vi "ARCH_AUDIT_EDITOR_prepare_SELECT_statement.vi"(7 "nmb_of_top_rows (all)":i32, 8 "error_in":errorcluster) -> (0 "error_out":errorcluster, 3 "SELECT_statement":string)   [LabVIEW 2020]
uses:
  FGV/ARCH_AUDIT_EDITOR_records_display/FGV_ARCH_AUDIT_EDITOR_records_display.ctl
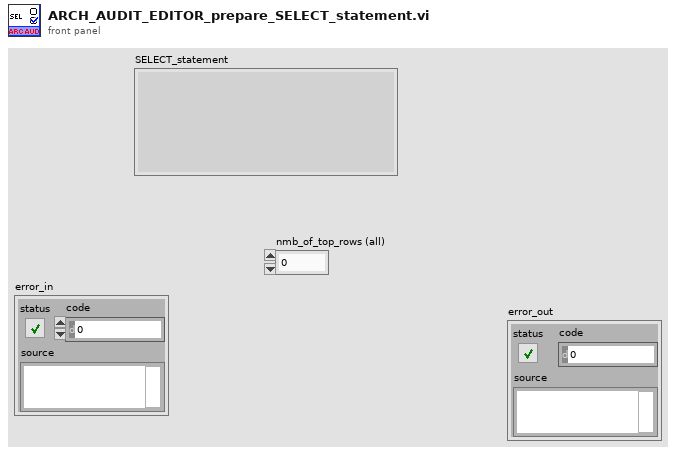
[diagram p1: front panel]
types:
  T1 = typedef "FGV_ARCH_AUDIT_EDITOR_records_display.ctl" = enum16{"initialize", "set_arch_cfg_tables_names", "set_station_number", "set_type_filter", "set_headers", "set_records", "get_arch_cfg_table_name", "get_arch_cfg_hist_table_name", "get_station_number", "get_type_filter", "get_headers", "get_uneditable_columns", "get_all_info", "record_added?", "record_inserted?", "record_edited?", "record_updated?", "record_deleted?", "discard_changes"}
  T2 = typedef "ARCH_AUDIT_EDITOR_all_info.ctl" = cluster{"station_number":string, "type_filter":string, "archivisation_audit_cfg_table":string, "archivisation_audit_cfg_history":string, "column_names":string[], "uneditable_columns":string[], "uneditable_columns":i32[], "editable_columns":i32[], "values_in_database":string[][], "size":cluster{"columns":i32, "SQL_rows":i32, "disp_rows":i32}, "ARCH_AUDIT_record_states":T3[]}
  T3 = typedef "SQL_record_states.ctl" = enum16{"Equal", "Added", "Edited", "Deleted"}
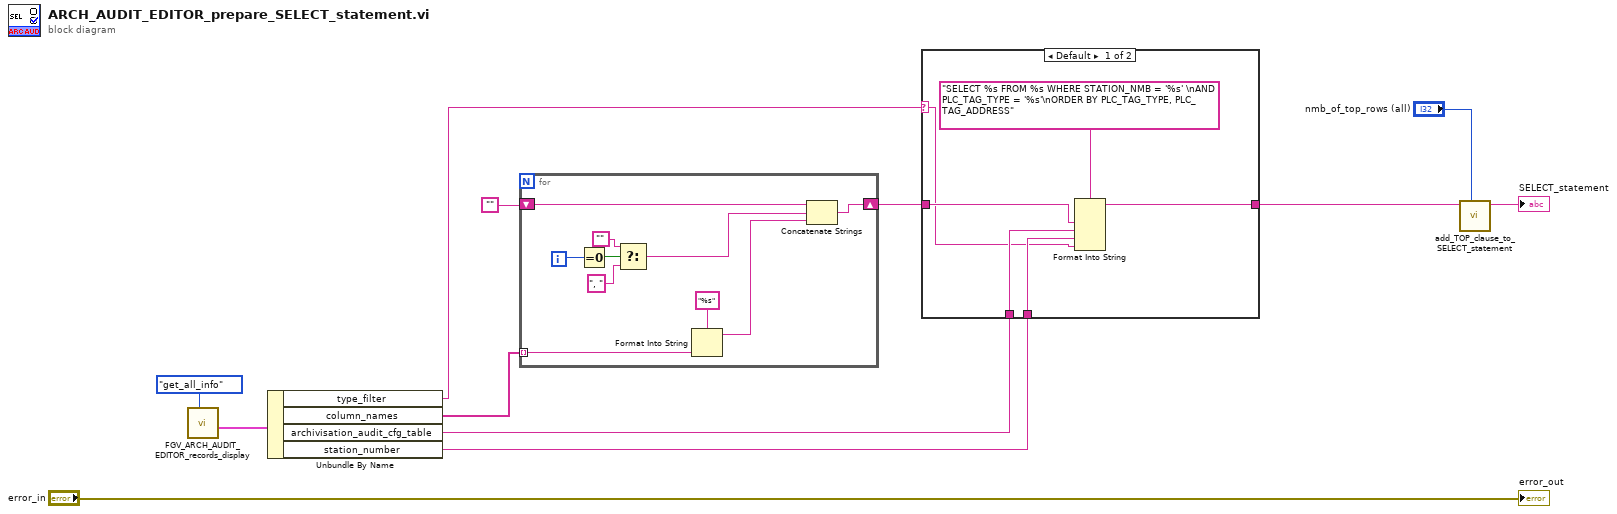
[diagram p0: block diagram]
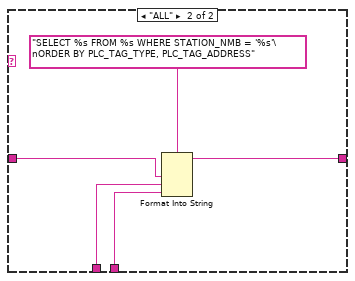
[diagram p2: hidden frame]
diagram:
  n1 = call "FGV_ARCH_AUDIT_EDITOR_records_display.vi"("options"=FGV_ARCH_AUDIT_EDITOR_records_display."get_all_info") -> ("all_info"=w5:T2)  [unwired: 7 in, 3 out]
  n2 = Unbundle By Name(w5) -> ("type_filter"=w7:string, "column_names"=w12:string[], "archivisation_audit_cfg_table"=w9:string, "station_number"=w8:string)
  n3 = for {
    tunnel: w12 -> [w15] mode=indexing
    shift-right: [w17] -> w10
    shift-left: "" -> [w18]
    i -> [w22]
    n4 = Equal To 0?(x=w22) -> (x = 0?=w21:bool)
    n5 = Select(t="", s=w21, f=", ") -> (s? t:f=w16:string)
    n6 = Format Into String(format string="%s", w15) -> (resulting string=w14:string)  [unwired: 2 in, 1 out]
    n7 = Concatenate Strings(w18, w16, w14) -> (w17:string)
  }
  n8 = case shown="Default" w7 {
    selector: w7 -> [w23 _]
    tunnel: w10 -> [w27 w32]
    tunnel: w9 -> [w25 w31]
    tunnel: w8 -> [w24 w30]
    tunnel: [w26 w29] -> w3
    frame Default {
      n9 = Format Into String(format string="SELECT %s FROM %s WHERE STATION_NMB = '%s' \nAND PLC_TAG_TYPE = '%s'\nORDER BY PLC_TAG_TYPE, PLC_TAG_ADDRESS", w27, w25, w24, w23) -> (resulting string=w26:string)  [unwired: 2 in, 1 out]
    }
    frame "ALL" {
      n10 = Format Into String(format string="SELECT %s FROM %s WHERE STATION_NMB = '%s'\nORDER BY PLC_TAG_TYPE, PLC_TAG_ADDRESS", w32, w31, w30) -> (resulting string=w29:string)  [unwired: 2 in, 1 out]
    }
  }
  n11 = call "add_TOP_clause_to_SELECT_statement.vi"("nmb_of_top_rows (all)"="nmb_of_top_rows (all)", "SELECT_statement_in"=w3) -> ("SELECT_statement_out"=→"SELECT_statement":string)  [unwired: 8 in, 1 out]
  "error_out" <- "error_in"
